vi "Compute Optimal Transition Time.vi"(8 "error in (no error)":errorcluster, 10 "optimum":T1, 11 "SV Multitone in":refnum<class "SV Multitone.lvclass">) -> (0 "error out":errorcluster, 2 "optimal transition time":dbl, 3 "SV Multitone out":refnum<class "SV Multitone.lvclass">)   [LabVIEW 2017, in "SV Multitone.lvclass"]
uses:
  <vilib>/addons/_NISVFA/_Generation/Signal Generation/SV Multitone/SV Multitone.lvclass
  <vilib>/addons/_NISVFA/_Generation/subVIs/sv_Optimum Location.ctl
  <vilib>/addons/_NISVFA/_Generation/Signal Generation/SV Multitone/SV Multitone.lvclass/SV Multitone.ctl
  <vilib>/addons/_NISVFA/_Generation/SoundVib_Generation.lvlib
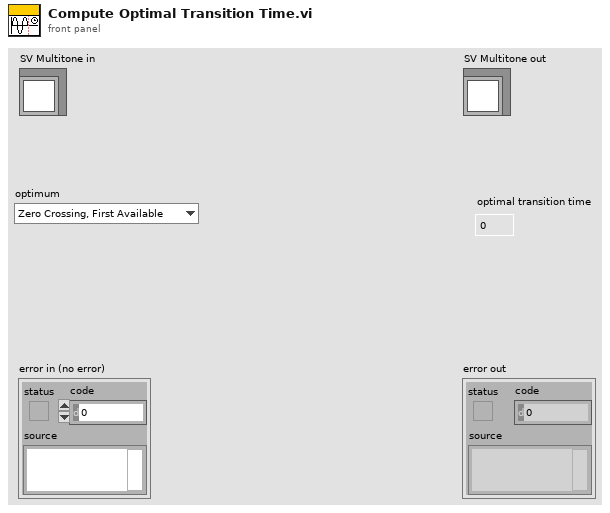
[diagram p1: front panel]
types:
  T1 = typedef "SoundVib_Generation.lvlib/sv_Optimum Location.ctl" = enum16{"Zero Crossing, First Available", "Zero Crossing, Positive Slope", "Zero Crossing, Negative Slope", "Peak or Valley", "Peak", "Valley"}
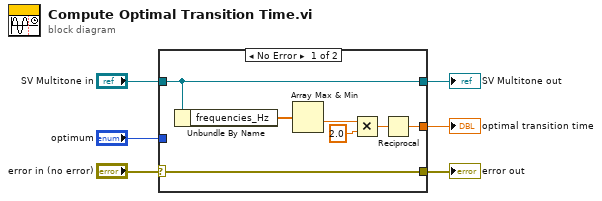
[diagram p0: block diagram]
diagram:
  n1 = case shown="No Error" "error in (no error)" {
    selector: "error in (no error)" -> [w8 w14]
    tunnel: "SV Multitone in" -> [w7 w15]
    tunnel: [w9 _] -> w5
    tunnel: [w8 w14] -> w3
    tunnel: [w7 w15] -> w2
    tunnel: "optimum" -> [_ _]
    frame No Error {
      n2 = Unbundle By Name(w7) -> ("frequencies_Hz"=w13:dbl[])
      n3 = Array Max & Min(array=w13) -> (min value=w12:dbl)  [unwired: 3 out]
      n4 = Multiply(x=w12, y=2.0) -> (x*y=w10:dbl)
      n5 = Reciprocal(x=w10) -> (1/x=w9:dbl)
    }
    frame Error {
    }
  }
  "error out" <- w3
  "SV Multitone out" <- w2
  "optimal transition time" <- w5
